vi "Day08-03_온도 센서.vi"(8 "error in":errorcluster caption="에러 입력") -> (0 "error out":errorcluster caption="에러 출력", 3 "task out":refnum<k21> caption="태스크 출력")   [LabVIEW 2021]
uses:
  <vilib>/DAQmx/create/channels.llb/DAQmx Create Channel (AI-Temperature-Thermocouple).vi
  <vilib>/DAQmx/configure/timing.llb/DAQmx Timing (Sample Clock).vi
  <resource>/objmgr/daqmx.rc
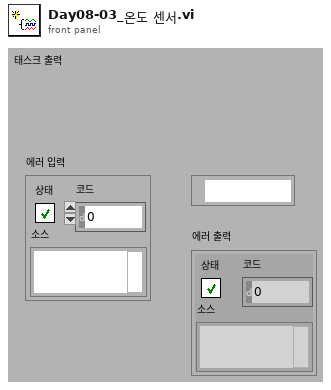
[diagram p1: front panel]
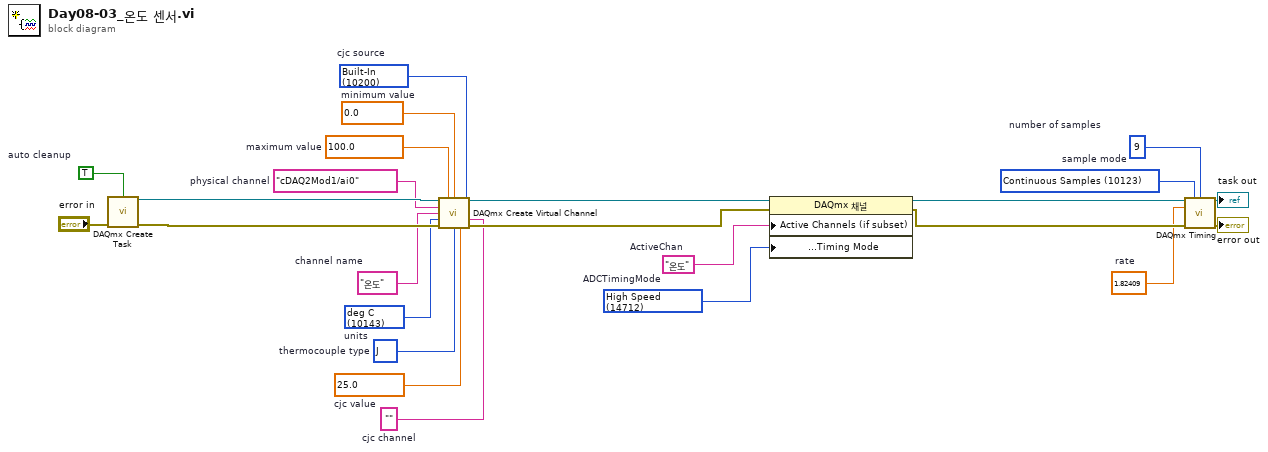
[diagram p0: block diagram]
diagram:
  w1 = 10123 items=["Finite Samples"=10178, "Continuous Samples"=10123, "Hardware Timed Single Point"=12522]  # sample mode
  w2 = 9  # number of samples
  w3 = 1.82409  # rate
  w7 = 14712 items=["Automatic"=16097, "High Resolution"=10195, "High Speed"=14712, "Best 50 Hz Rejection"=14713, "Best 60 Hz Rejection"=14714, "Custom"=10137]  # ADCTimingMode
  w10 = "온도"  # ActiveChan
  w11 = 10200 items=["Built-In"=10200, "Constant Value"=10116, "Channel"=10113]  # cjc source
  w13 = ""  # cjc channel
  w14 = 25.0  # cjc value
  w15 = 10072 items=["J"=10072, "K"=10073, "N"=10077, "R"=10082, "S"=10085, "T"=10086, "B"=10047, "E"=10055]  # thermocouple type
  w16 = 10143 items=["deg C"=10143, "deg F"=10144, "Kelvins"=10325, "deg R"=10145, "From Custom Scale"=10065]  # units
  w12 = "온도"  # channel name
  w18 = 0.0  # minimum value
  w19 = 100.0  # maximum value
  w20 = "cDAQ2Mod1/ai0"  # physical channel
  w22 = TRUE  # auto cleanup
  n1 = call <vilib>:"DAQmx Create Task.vi"("auto cleanup"=w22, "error in"="error in") -> ("task out"=w21:refnum<k21>, "error out"=w23:errorcluster)  [unwired: 12 in]
  n2 = call-poly <vilib>:"DAQmx Create Virtual Channel.vi"("task in"=w21, "maximum value"=w19, "minimum value"=w18, "physical channels"=w20, "cjc source"=w11, "name to assign"=w12, "units"=w16, "cjc channel"=w13, "error in"=w23, "thermocouple type"=w15, "cjc value"=w14) -> ("task out"=w8:refnum<k21>, "error out"=w17:errorcluster)  [unwired: 3 in]
  n3 = property class="DAQmx 채널"(reference=w8, error in=w17, "Active Channels (if subset)"=w10, "Analog Input:General Properties:Digitizer/ADC:Timing Mode"=w7) -> (reference out=w4:refnum<k21>, error out=w9:errorcluster)
  n4 = call-poly <vilib>:"DAQmx Timing.vi"("task/channels in"=w4, "sample mode"=w1, "samples per channel"=w2, "rate"=w3, "error in"=w9) -> ("task out"=→"task out":refnum<k21>, "error out"=→"error out":errorcluster)  [unwired: 9 in]
